vi "Test Synapse Read Waves.vi"() -> ()   [LabVIEW 2015]
uses:
  PXI DAQ VIs/Utility VIs/Array Dimensions (2D).vi
panel:
  out "Array 2":i32[][](array[numeric])
  out "Array":i32[](array[numeric])
  in  "stop":bool
  out "Graph":dbl[][](graph)
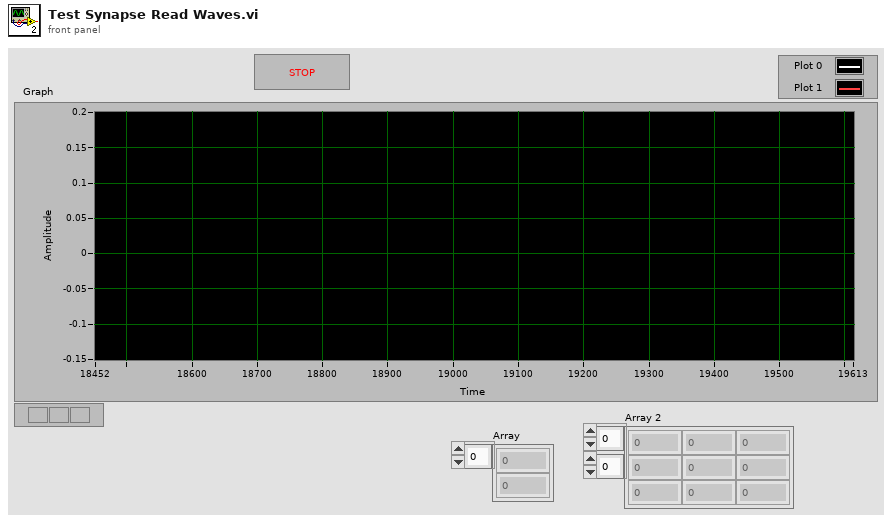
[diagram p1: front panel]
types:
  T1 = typedef "TDTSyn-Settings.ctl" = cluster{"Server IP Address":u32, "TCP Port":u16, "Synapse URL":string, "Tank Root":string}
  T2 = typedef "TDTSyn-State.ctl" = cluster{"TTankX":refnum<k7>, "LastTime":dbl[], "error":errorcluster, "Block Name":string, "Tank Name":string, "NumTicks":i32, "LastTick":dbl[], "LastArtf":dbl, "ChanCount":i32[], "TickSource":i32, "Tank Codes":string[], "waves Tlast":dbl}
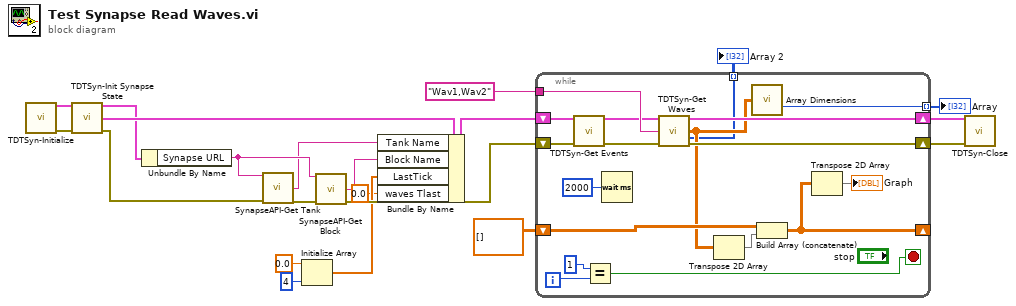
[diagram p0: block diagram]
diagram:
  n1 = call "TDTSyn-Initialize.vi"() -> ("Settings"=w20:T1, "error out"=w21:errorcluster)  [unwired: 14 in]
  n2 = call "TDTSyn-Init Synapse State.vi"("Settings"=w20, "error in (no error)"=w21) -> ("Settings (thru)"=w15:T1, "State"=w19:T2, "error out"=w14:errorcluster)  [unwired: 11 in]
  n3 = Unbundle By Name(w15) -> ("Synapse URL"=w13:string)
  n4 = call "SynapseAPI-Get Tank.vi"("URL"=w13, "error in (no error)"=w14) -> ("tank"=w11:string, "error out"=w16:errorcluster)  [unwired: 12 in]
  n5 = Initialize Array(0.0 ("element"), 4 ("dimension size")) -> (w4:dbl[])
  n6 = call "SynapseAPI-Get Block.vi"("URL"=w13, "error in (no error)"=w16) -> ("block"=w10:string, "error out"=w9:errorcluster)  [unwired: 12 in]
  n7 = Bundle By Name(cluster=w19, "Tank Name"=w11, "Block Name"=w10, "LastTick"=w4, "waves Tlast"=0.0) -> (w12:T2)
  n8 = while {
    tunnel: "Wav1,Wav2" ("codes") -> [w37]
    shift-right: [w39] -> w18
    shift-left: w12 -> [w34]
    shift-right: [w38] -> w17
    shift-left: w9 -> [w35]
    shift-right: [w26] -> _
    shift-left: dbl[][] [] -> [w31]
    tunnel: [w23] -> w3 mode=indexing
    tunnel: [w22] -> w2 mode=indexing
    i -> [w30]
    stop <- w28 stop-if-true
    n9 = call "TDTSyn-Get Events.vi"("State In"=w34, "error in (no error)"=w35) -> ("State Out"=w33:T2, "error out"=w32:errorcluster)  [unwired: 10 in, 2 out]
    n10 = Equal?(x=1, y=w30) -> (x = y?=w28:bool)
    n11 = Wait (ms)(milliseconds to wait=u32 2000) -> ()  [unwired: 1 out]
    n12 = call "TDTSyn-Get Waves.vi"("State In"=w33, "codes"=w37, "error in (no error)"=w32) -> ("State Out"=w39:T2, "Waves"=w24:dbl[][], "Array"=w22:i32[], "error out"=w38:errorcluster)  [unwired: 9 in]
    n13 = Transpose 2D Array(2D array=w24) -> (transposed array=w27:dbl[][])
    n14 = call-poly "Array Dimensions.vi"("2D Array"=w24) -> ("# columns"=w23:i32)  [unwired: 13 in, 1 out]
    n15 = Build Array (concatenate)(w31, w27) -> (w26:dbl[][])
    n16 = Transpose 2D Array(2D array=w26) -> (transposed array=→"Graph":dbl[][])
  }
  "Array" <- w3
  "Array 2" <- w2
  n17 = call "TDTSyn-Close.vi"("State in"=w18, "error in (no error)"=w17) -> ()  [unwired: 12 in, 2 out]
